vi "savePNG.vi"(8 "error in":errorcluster, 10 "image path in (.bmp)":path, 11 "controls array in":refnum<vi>[](array[refnum])) -> (0 "error out":errorcluster, 2 "image path out (.PNG)":path, 3 "controls array out":refnum<vi>[](array[refnum]))   [LabVIEW 2019]
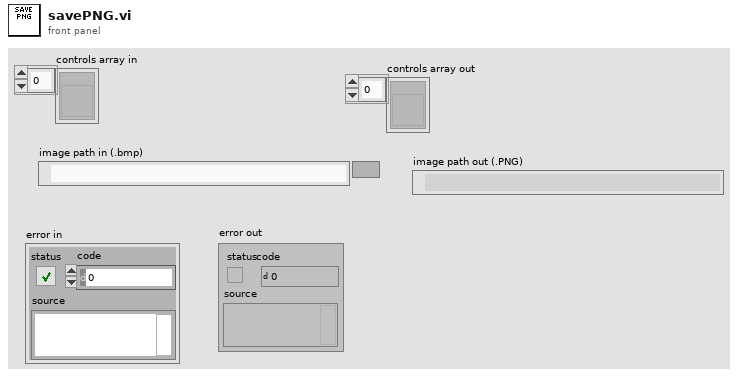
[diagram p1: front panel]
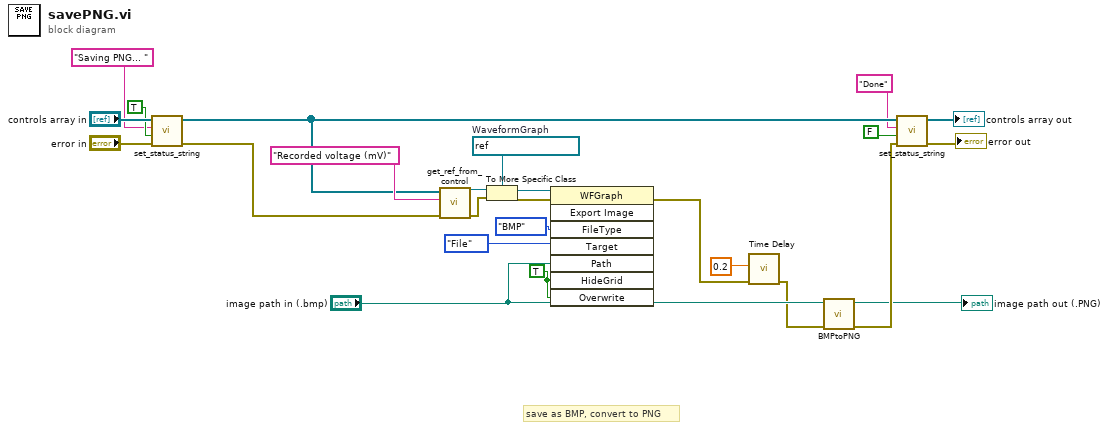
[diagram p0: block diagram]
diagram:
  w18 = TRUE ("Hide Grid")
  w22 = refnum<vi> refnum  # WaveformGraph
  # "save as BMP, convert to PNG"
  n1 = call "set_status_string.vi"("error in"="error in", "new line?"=TRUE, "status string in"="Saving PNG... ", "controls array"="controls array in") -> ("error out"=w8:errorcluster, "controls array out"=w7:refnum<vi>[])  [unwired: 6 in]
  n2 = call "get_ref_from_control.vi"("error in"=w8, "control label"="Recorded voltage (mV)", "controls array"=w7) -> ("error out"=w24:errorcluster, "reference out"=w23:refnum<vi>)  [unwired: 7 in]
  n3 = To More Specific Class(target class=w22, reference=w23, error in=w24) -> (specific class reference=w21:refnum<vi>, error out=w19:errorcluster)
  n4 = invoke class="WFGraph" method="Export Image"(reference=w21, error in=w19, "FileType"=enum32{"BMP", "EPS", "EMF", "PICT"}."BMP" ("File Type"), "Target"=enum32{"File", "Clipboard"}."File", "Path"="image path in (.bmp)", "HideGrid"=w18, "Overwrite"=w18) -> (error out=w15:errorcluster)  [unwired: 1 in, 7 out]
  n5 = call "Time Delay"("error in (no error)"=w15, "Delay Time (s)"=0.2) -> ("error out"=w14:errorcluster)  [unwired: 9 in]
  n6 = call "BMPtoPNG.vi"("error in"=w14, "image path in (.bmp)"="image path in (.bmp)") -> ("error out"=w4:errorcluster, "image path out (.png)"=→"image path out (.PNG)":path)  [unwired: 8 in]
  n7 = call "set_status_string.vi"("error in"=w4, "new line?"=FALSE, "status string in"="Done", "controls array"=w7) -> ("error out"=→"error out":errorcluster, "controls array out"=→"controls array out":refnum<vi>[])  [unwired: 6 in]
